vi "sync and trig.vi"(8 "error in (no error)":errorcluster, 10 "time calibrate":dbl[](array[numeric]), 11 "5785_3.2GHz_one channel in":refnum<class "5785_3.2GHz_one channel.lvclass">) -> (0 "error out":errorcluster, 3 "5785_3.2GHz_one channel out":refnum<class "5785_3.2GHz_one channel.lvclass">)   [LabVIEW 2021, in "5785_3.2GHz_one channel.lvclass"]
uses:
  5785_3.2GHz_one channel.lvclass
  5785_3.2GHz_one channel.lvclass/5785_3.2GHz_one channel.ctl
  <vilib>/Utility/error.llb/Error Cluster From Error Code.vi
  <vilib>/rvi/errors/niLvFpgaAdjustHostInterfaceError.vi
  <instrlib>/_niInstr/Streaming/v1/Host/Public/Start Continuous Stream.vi
  <vilib>/rvi/interface/nirviReadWriteControl/nirviReadWriteControl.xnode
  <instrlib>/_niInstr/Streaming/v1/Host/niInstr Streaming v1 Host.lvlib
  <resource>/objmgr/sessionReference.rc
  NiFpgaLv.dll
  <vilib>/rvi/interface/Simulation/niFpgaSimulationCallBeginRW.vi
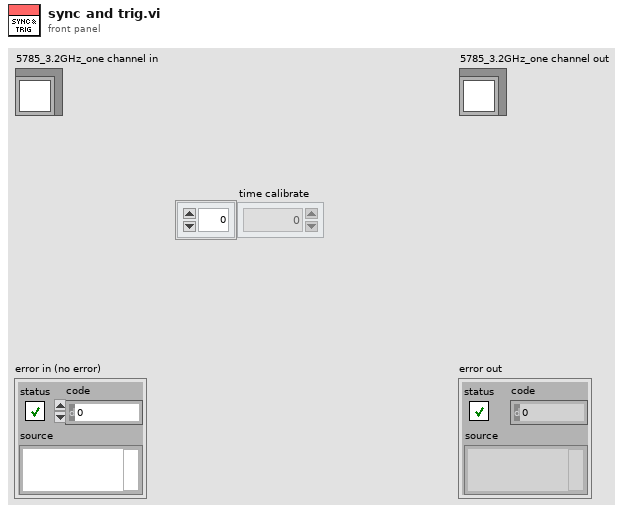
[diagram p1: front panel]
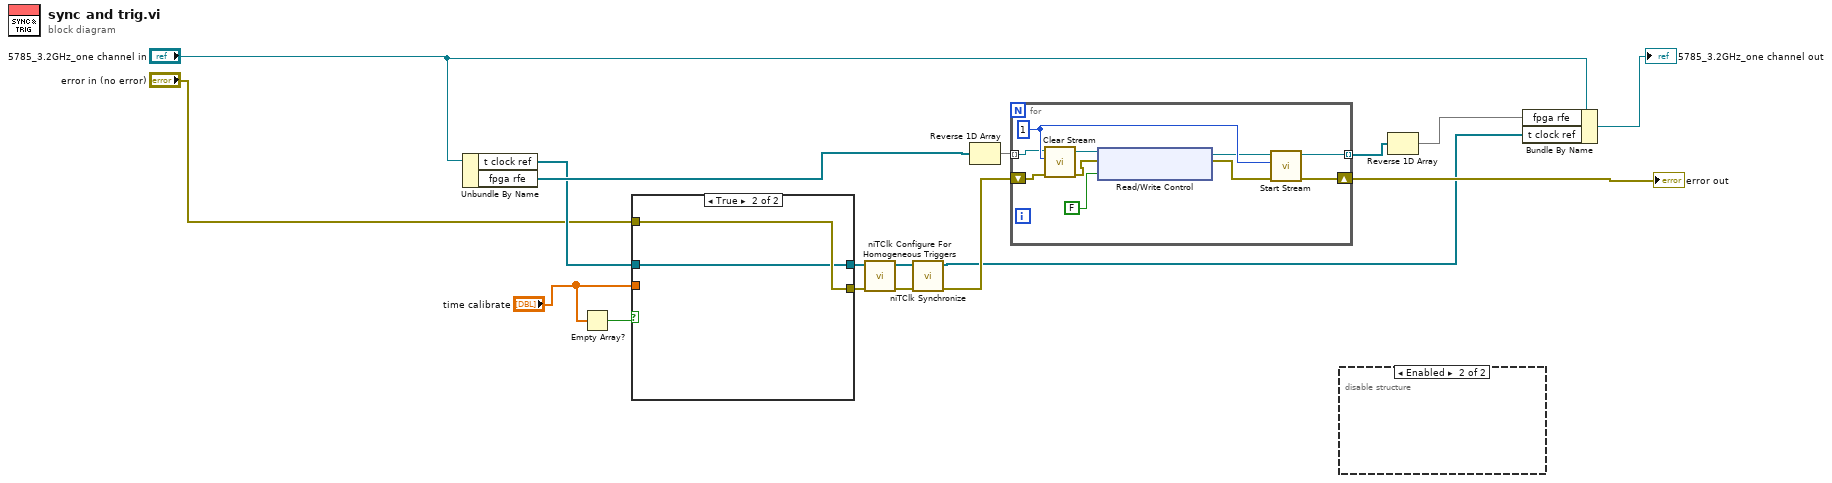
[diagram p0: block diagram]
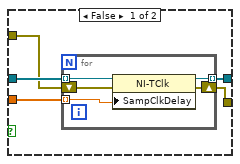
[diagram p2: hidden frame]
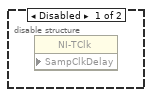
[diagram p3: hidden frame]
diagram:
  n1 = Unbundle By Name("5785_3.2GHz_one channel in") -> ("t clock ref"=w8:refnum<k20>[], "fpga rfe"=w13:refnum<k20>[])
  n2 = Empty Array?(array="time calibrate") -> (empty?=w1:bool)
  n3 = case shown="True" w1 {
    tunnel: w8 -> [w22 w28]
    tunnel: [w21 w28] -> w7
    tunnel: "error in (no error)" -> [w20 w29]
    tunnel: [w19 w29] -> w5
    tunnel: "time calibrate" -> [w18 _]
    frame False {
      n4 = for {
        tunnel: w22 -> [w27] mode=indexing
        tunnel: [w26] -> w21 mode=indexing
        shift-right: [w24] -> w19
        shift-left: w20 -> [w25]
        tunnel: w18 -> [w23] mode=indexing
        n5 = property class="NI-TClk"(reference=w27, error in=w25, "SampClkDelay"=w23) -> (reference out=w26:refnum<k20>, error out=w24:errorcluster)
      }
    }
    frame True {
    }
  }
  n6 = call <instrlib>:"niTClk Configure For Homogeneous Triggers.vi"("error in (no error)"=w5, "sessions"=w7) -> ("error out"=w14:errorcluster, "sessions out"=w15:refnum<k20>[])  [unwired: 8 in]
  n7 = call <instrlib>:"niTClk Synchronize.vi"("error in (no error)"=w14, "sessions"=w15) -> ("error out"=w17:errorcluster, "sessions out"=w10:refnum<k20>[])  [unwired: 8 in]
  n8 = Reverse 1D Array(array=w13) -> (reversed array=w16:refnum<k20>[])
  n9 = for {
    tunnel: w16 -> [w35] mode=indexing
    shift-right: [w38] -> w12
    shift-left: w17 -> [w34]
    tunnel: [w37] -> w4 mode=indexing
    w39 = 1 ("stream index")
    n10 = call <instrlib>:"Clear Stream.vi"("error in (no error)"=w34, "stream index"=w39, "refnum in"=w35) -> ("error out"=w33:errorcluster, "refnum out"=w32:refnum<k20>)  [unwired: 7 in]
    n11 = xnode "Read/Write Control"("FPGA VI Reference In"=w32, "error in"=w33, "reset system clock"=FALSE) -> ("FPGA VI Reference Out"=w30:refnum<k20>, "error out"=w31:errorcluster)
    n12 = call-poly <instrlib>:"Start Stream.vi"("error in (no error)"=w31, "stream index"=w39, "refnum in"=w30) -> ("error out"=w38:errorcluster, "refnum out"=w37:refnum<k20>)  [unwired: 7 in]
  }
  "error out" <- w12
  n13 = disable-structure shown="Enabled" {
    frame Disabled {
      n14 = property class="NI-TClk" props=["SampClkDelay"]() -> ()  [unwired: 3 in, 2 out]
    }
    frame Enabled {
    }
  }
  n15 = Reverse 1D Array(array=w4) -> (reversed array=w3:refnum<k20>[])
  n16 = Bundle By Name(cluster="5785_3.2GHz_one channel in", "fpga rfe"=w3, "t clock ref"=w10) -> (→"5785_3.2GHz_one channel out":refnum<class "5785_3.2GHz_one channel.lvclass">)
